vi "Color Comparison.vi"(8 "error in (no error)":errorcluster, 9 "Setpoint":dbl=1.0, 10 "Level":dbl, 11 "C100L in":refnum<class "C100L.lvclass">) -> (0 "error out":errorcluster, 2 "Color":u32(colorbox))   [LabVIEW 2021, in "C100L.lvlib" / "C100L.lvclass"]
uses:
  C100L.lvclass
  C100L.lvclass/C100L.ctl
  <vilib>/NathanCo/Color Compare/Percent Difference/Percent Difference.lvclass
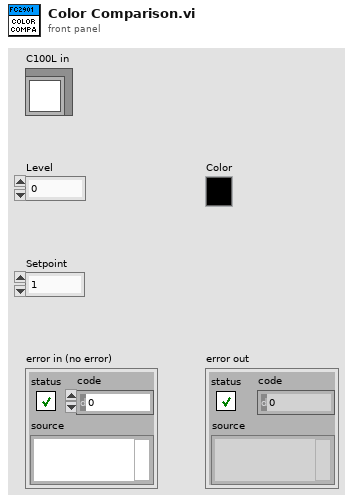
[diagram p1: front panel]
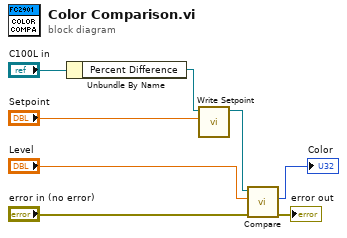
[diagram p0: block diagram]
diagram:
  n1 = Unbundle By Name("C100L in") -> ("Percent Difference"=w6:refnum<class "Percent Difference.lvclass">)
  n2 = call <vilib>:"Write Setpoint.vi"("Setpoint"="Setpoint", "Percent Difference in"=w6) -> ("Percent Difference out"=w5:refnum<class "Percent Difference.lvclass">)  [unwired: 8 in, 1 out]
  n3 = call-dynamic "Compare.vi"("error in (no error)"="error in (no error)", "Level"="Level", "Percent Difference in"=w5) -> ("error out"=→"error out":errorcluster, "Color"=→"Color":u32)  [unwired: 7 in]
